vi "Build Basic Bus Monitor.vi"(6 "48-bit Time Tag":bool, 8 "error in (no error)":errorcluster, 11 "1553 Test in":refnum<class "1553 Test.lvclass">) -> (0 "error out":errorcluster, 3 "1553 Test out":refnum<class "1553 Test.lvclass">)   [LabVIEW 2016, in "1553 Test.lvclass"]
uses:
  1553 Test.lvclass
  Bus Monitor/Bus Monitor.lvclass
  Bus Monitor/TypeDefs/Bus Monitor Configuration.ctl
  1553 Component/1553 Component.lvclass
  Filters/Filter/Filter.lvclass
  Frames & Messages/TypeDefs/Command Type.ctl
  BCI-1553 API.lvlib
  Filters/TypeDefs/Filter Configuration.ctl
  Bus Monitor/TypeDefs/Bus Monitor Timetag Configuration.ctl
  Bus Monitor/TypeDefs/Bus Monitor Record Requirement.ctl
  Bus Monitor/TypeDefs/Bus Monitor Timetag Behavior.ctl
  Bus Monitor/TypeDefs/Bus Monitor Timeout.ctl
  D:/R&D/cRIO 1553 2016/Windows/1553 SubComponent/1553 SubComponent.lvclass
  Dependencies/FPGA Interface/FPGA Interface.lvclass
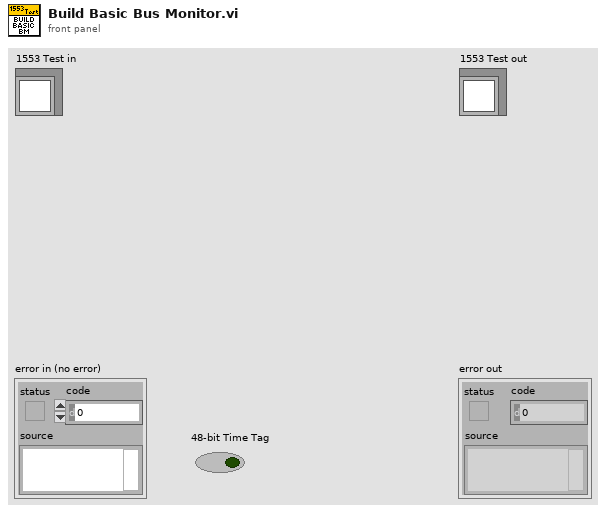
[diagram p1: front panel]
types:
  T1 = typedef "BCI-1553 API.lvlib/Filter Configuration.ctl" = cluster{"Filter Type":T2, "Terminal Address (0-30)":u16, "SubAddress (1-30)":u16, "Mode Code":bool, "Broadcast":bool, "RT-RT":bool, "Bus A":bool}
  T2 = typedef "BCI-1553 API.lvlib/Command Type.ctl" = enum16{"Transmit", "Receive"}
  T3 = typedef "BCI-1553 API.lvlib/Bus Monitor.lvclass/Bus Monitor Configuration.ctl" = cluster{"Timeout":T4, "Gap Check":bool, "Timetag Behavior":T5, "Record Requirement":T6, "Cont Record After Inv Word":bool, "Ext Msg Flag Enable":bool, "48-bit Time Tag":bool, "Simple Mode":bool, "Bus Monitor Timetag Config":T7}
  T4 = typedef "BCI-1553 API.lvlib/Bus Monitor.lvclass/Bus Monitor Timeout.ctl" = enum16{"18us", "23us", "82us", "140us"}
  T5 = typedef "BCI-1553 API.lvlib/Bus Monitor.lvclass/Bus Monitor Timetag Behavior.ctl" = enum16{"Last Bit of Last Word", "First Bit of Command Word", "Last Bit of Command Word", "Timetag Disabled"}
  T6 = typedef "BCI-1553 API.lvlib/Bus Monitor.lvclass/Bus Monitor Record Requirement.ctl" = enum16{"Properly Encoded - Complete - Cmd Sync", "Properly Encoded - Complete - Cmd or Data Sync", "Properly Encoded Cmd Sync - At Least 2 Data Bits ", "Any Properly Encoded Sync - At Least 2 Data Bits"}
  T7 = typedef "BCI-1553 API.lvlib/Bus Monitor.lvclass/Bus Monitor Timetag Configuration.ctl" = enum16{"Disabled", "2us", "4us", "8us", "16us", "32us", "64us", "100ns"}
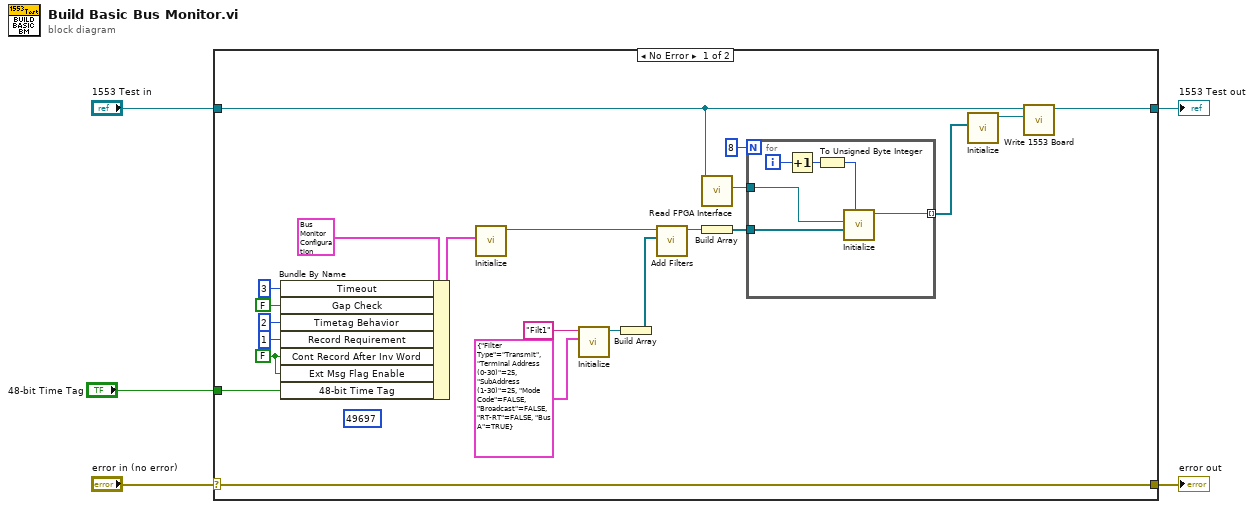
[diagram p0: block diagram]
diagram:
  n1 = case shown="No Error" "error in (no error)" {
    selector: "error in (no error)" -> [w27 w35]
    tunnel: [w27 w35] -> w4
    tunnel: [w20 w34] -> w2
    tunnel: "1553 Test in" -> [w21 w34]
    tunnel: "48-bit Time Tag" -> [w17 _]
    frame No Error {
      (unwired) u16 49697
      w16 = FALSE ("Cont Record After Inv Word")
      n2 = Bundle By Name(cluster=T3 {"Timeout"=enum."18us", "Gap Check"=FALSE, "Timetag Behavior"=enum."Last Bit of Last Word", "Record Requirement"=enum."Properly Encoded - Complete - Cmd Sync", "Cont Record After Inv Word"=FALSE, "Ext Msg Flag Enable"=FALSE, "48-bit Time Tag"=FALSE, "Simple Mode"=FALSE, "Bus Monitor Timetag Config"=enum."Disabled"} ("Bus Monitor Configuration"), "Timeout"=u8 3 ("BM Timeout"), "Gap Check"=FALSE, "Timetag Behavior"=u8 2 ("BM Time Tag Msg Bit Select"), "Record Requirement"=u8 1 ("BM Start Record Req"), "Cont Record After Inv Word"=w16, "Ext Msg Flag Enable"=w16, "48-bit Time Tag"=w17) -> (w18:T3)
      n3 = call "Initialize.vi"("Bus Monitor Configuration"=w18) -> ("Bus Monitor out"=w11:refnum<class "Bus Monitor.lvclass">)  [unwired: 9 in, 1 out]
      n4 = call "Initialize.vi"("Filter Configuration"=T1 {"Filter Type"=enum."Transmit", "Terminal Address (0-30)"=25, "SubAddress (1-30)"=25, "Mode Code"=FALSE, "Broadcast"=FALSE, "RT-RT"=FALSE, "Bus A"=TRUE}, "ID"="Filt1") -> ("Filter out"=w9:refnum<class "Filter.lvclass">)  [unwired: 8 in, 1 out]
      n5 = Build Array(w9) -> (w8:refnum<class "Filter.lvclass">[])
      n6 = call-dynamic "Add Filters.vi"("Filters"=w8, "Bus Monitor in"=w11) -> ("Bus Monitor out"=w10:refnum<class "Bus Monitor.lvclass">)  [unwired: 8 in, 1 out]
      n7 = call-dynamic "Read FPGA Interface.vi"("1553 Test in"=w21) -> ("FPGA Interface"=w23:refnum<class "FPGA Interface.lvclass">)  [unwired: 8 in, 2 out]
      n8 = Build Array(w10) -> (w24:refnum<class "Bus Monitor.lvclass">[])
      n9 = for {
        N: 8 -> [_]
        tunnel: [w31] -> w25 mode=indexing
        tunnel: w24 -> [w30]
        tunnel: w23 -> [w29]
        i -> [w33]
        n10 = Increment(x=w33) -> (x+1=w28:i32)
        n11 = To Unsigned Byte Integer(number=w28) -> (unsigned 8bit integer=w32:u8)
        n12 = call "Initialize.vi"("Component ID (1-8)"=w32, "SubComponents"=w30, "FPGA Interface"=w29) -> ("1553 Component out"=w31:refnum<class "1553 Component.lvclass">)  [unwired: 7 in, 1 out]
      }
      n13 = call "Initialize.vi"("Components"=w25) -> ("1553 Board out"=w26:refnum<class "1553 Board.lvclass">)  [unwired: 9 in, 1 out]
      n14 = call-dynamic "Write 1553 Board.vi"("1553 Board"=w26, "1553 Test in"=w21) -> ("1553 Test out"=w20:refnum<class "1553 Test.lvclass">)  [unwired: 8 in, 1 out]
    }
    frame Error {
    }
  }
  "error out" <- w4
  "1553 Test out" <- w2
